vi "ni5660 Fetch IQ.vi"(0 "receiver info in":T1, 5 "samples to read":i32=-1, 7 "timeout (sec)":dbl=5.0 format="%.2f", 11 "error in (no error)":errorcluster) -> (4 "receiver info out":T1, 6 "IQ waveform":cluster{"t0":dbl, "dt":dbl, "Y":cdb[]} {"Y" format="%.2f"; "dt" format="%.2f"; "t0" format="%.2f"}, 15 "error out":errorcluster)   [LabVIEW 2011]
doc: "This VI returns the IQ waveform acquired by the RF Signal Analyzer during a previously initiated acquisition. This VI returns IQ data computed through a process of filtering, decimation, and downconversion. Use this VI with the ni5660 Initiate VI when continuously acquiring data. \n\n<B>Note</B> Continous IQ acquisition is only possible for bandwidths smaller than 1.25 MHz."
uses:
  <vilib>/addons/Modulation/niScope/controls/mod_Modulation Settings.ctl
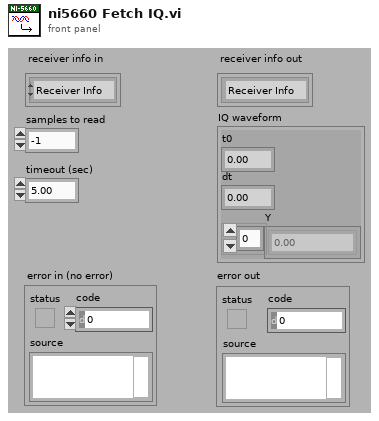
[diagram p1: front panel]
types:
  T1 = typedef "mod_Modulation Settings.ctl" = cluster{enum16{"Receiver Info"}, variant}
  T2 = enum16{"V", "V^2", "W", "dBm", "dBW", "dBV", "dBmV", "dBuV"}
  T3 = typedef "mod_Readable Attributes Cluster.ctl" = cluster{"carrier":cluster{"frequency":dbl}, "receiver":cluster{"handles":cluster{"niTuner taskID":i32, "niScope handle":refnum<k15>}, "RFSA":cluster{"reference level":i32, "RF attenuation":i32}, "data format":enum16{"real", "complex modulated (array)", "complex modulated (interleaved)"}, "auto suppress SW IQ":enum16{"off", "on"}, "IQ sample rate":dbl, "bandwidth":dbl}}
  T4 = cluster{"relativeInitialX":dbl, "xIncrement":dbl, "wfm":dbl[]}
  T5 = cluster{"actualSamples":i32, "absoluteInitialX":dbl, "relativeInitialX":dbl, "xIncrement":dbl, "offset":dbl, "gain":dbl, "reserved1":dbl, "reserved2":dbl}
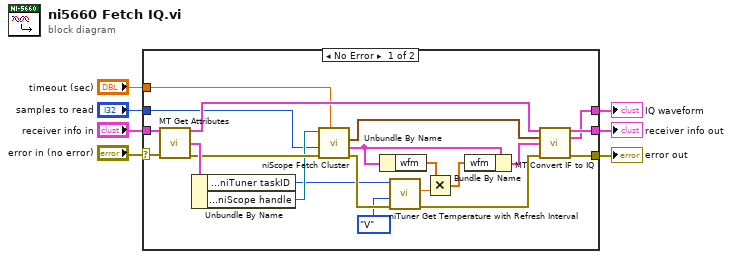
[diagram p0: block diagram]
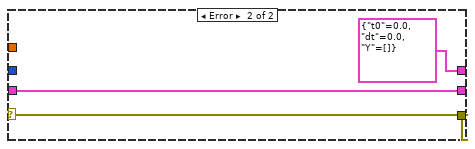
[diagram p2: hidden frame]
diagram:
  n1 = case shown="No Error" "error in (no error)" {
    selector: "error in (no error)" -> [w20 w31]
    tunnel: [w14 w31] -> w7
    tunnel: [w15 w30] -> w2
    tunnel: "receiver info in" -> [w19 w30]
    tunnel: "samples to read" -> [w13 _]
    tunnel: "timeout (sec)" -> [w12 _]
    tunnel: [w11 cluster{"t0":dbl, "dt":dbl, "Y":cdb[]} {"t0"=0.0, "dt"=0.0, "Y"=[]} ("IQ data (complex)")] -> w1
    frame No Error {
      n2 = call <vilib>:"MT Get Attributes.vi"("receiver info in"=w19, "error in (no error)"=w20) -> ("receiver info out"=w16:T1, "attributes"=w22:T3, "error out"=w21:errorcluster)  [unwired: 11 in]
      n3 = Unbundle By Name(w22) -> ("receiver.handles.niTuner taskID"=w17:i32, "receiver.handles.niScope handle"=w18:refnum<k15>)
      n4 = call <instrlib>:"niScope Fetch Cluster.vi"("timeout"=w12, "error in"=w21, "numSamples"=w13, "instrument handle"=w18) -> ("error out"=w28:errorcluster, "waveform"=w9:T4, "wfm info"=w23:T5)  [unwired: 4 in, 1 out]
      n5 = Unbundle By Name(w9) -> ("wfm"=w8:dbl[])
      n6 = call <instrlib>:"niTuner Get Temperature with Refresh Interval.vi"("error in"=w28, "correction units"=T2."V", "taskID in"=w17) -> ("error out"=w26:errorcluster, "correction factor"=w27:dbl)  [unwired: 5 in, 2 out]
      n7 = Multiply(x=w8, y=w27) -> (x*y=w25:dbl[])
      n8 = Bundle By Name(cluster=w9, "wfm"=w25) -> (w24:T4)
      n9 = call <vilib>:"MT Convert IF to IQ.vi"("receiver info in"=w16, "wfm info"=w23, "waveform in"=w24, "error in (no error)"=w26) -> ("receiver info out"=w15:T1, "IQ data (complex)"=w11:cluster{"t0":dbl, "dt":dbl, "Y":cdb[]}, "error out"=w14:errorcluster)  [unwired: 9 in]
    }
    frame Error {
    }
  }
  "error out" <- w7
  "receiver info out" <- w2
  "IQ waveform" <- w1
